vi "Drive for Time.vi"(8 "error in":errorcluster, 9 "Cluster":T6, 10 "Drivetrain":T1={"DevStatus"={"status"=FALSE, "code"=0, "source"=""}, "Motors[]"=[], "Square Inputs"=FALSE, "Max Output"=1.0}, 11 "Queue in":refnum<queue>) -> (0 "error out":errorcluster)   [LabVIEW 2016, in "Drive System.lvlib"]
uses:
  Drive System.lvlib
  DriveCmd.ctl
  DriveCmdList.ctl
  Varient Cmd Types/Drive Time.ctl
  <vilib>/Rock Robotics/WPI/RobotDrive/WPI_RobotDriveDevRef.ctl
  <vilib>/Rock Robotics/WPI/MotorControl/WPI_MotorControlDeviceRef.ctl
  <vilib>/Rock Robotics/WPI/MotorControl/WPI_MotorControlType.ctl
  <vilib>/Rock Robotics/SystemInterfaces/DIO/FPGA_DIOPWMChannel.ctl
  <vilib>/Rock Robotics/WPI/PWM/WPI_PWMDeadband.ctl
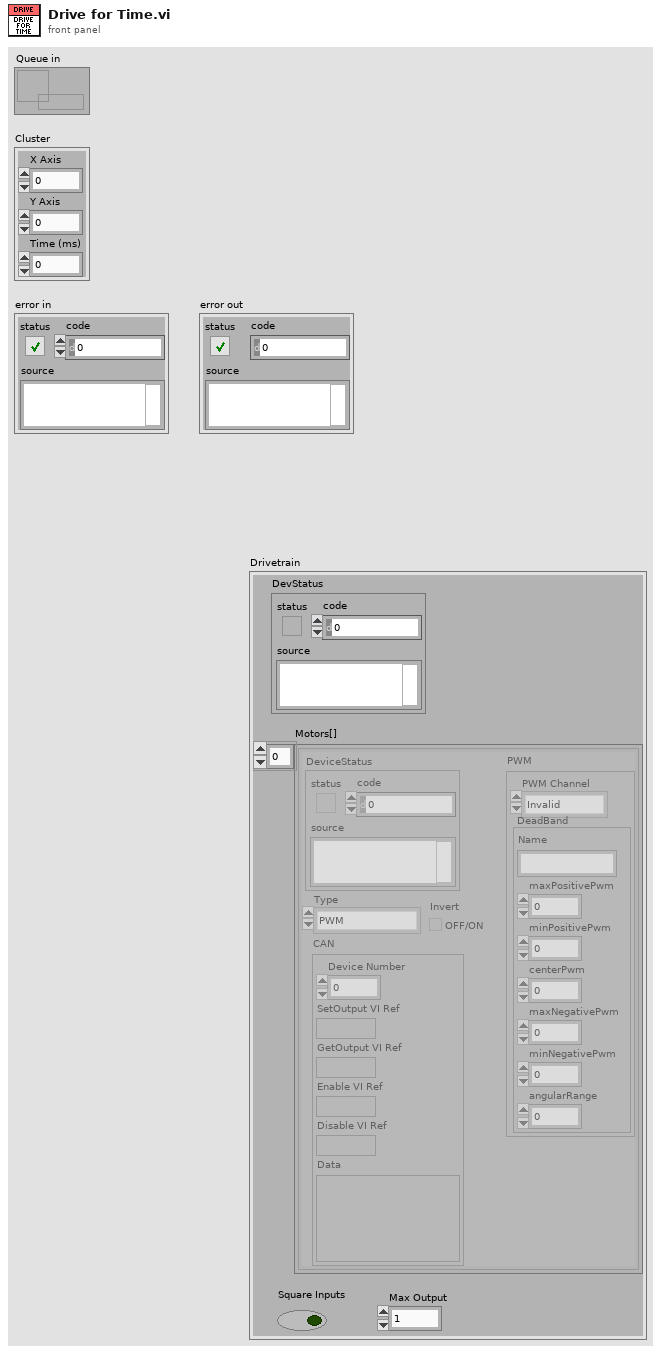
[diagram p1: front panel]
types:
  T1 = typedef "WPI_RobotDriveDevRef.ctl" = cluster{"DevStatus":errorcluster, "Motors[]":T2[], "Square Inputs":bool, "Max Output":dbl}
  T2 = typedef "WPI_MotorControlDeviceRef.ctl" = cluster{"DeviceStatus":errorcluster, "Type":T3, "PWM":cluster{"PWM Channel":T4, "DeadBand":T5}, "CAN":cluster{"Device Number":u8, "SetOutput VI Ref":variant, "GetOutput VI Ref":variant, "Enable VI Ref":variant, "Disable VI Ref":variant, "Data":variant}, "Invert":bool}
  T3 = typedef "WPI_MotorControlType.ctl" = enum16{"PWM", "CAN"}
  T4 = typedef "FPGA_DIOPWMChannel.ctl" = enum8{"PWM 0", "PWM 1", "PWM 2", "PWM 3", "PWM 4", "PWM 5", "PWM 6", "PWM 7", "PWM 8", "PWM 9", "PWM MXP 0", "PWM MXP 1", "PWM MXP 2", "PWM MXP 3", "PWM MXP 4", "PWM MXP 5", "PWM MXP 6", "PWM MXP 7", "PWM MXP 8", "PWM MXP 9", "Invalid"}
  T5 = typedef "WPI_PWMDeadband.ctl" = cluster{"Name":string, "maxPositivePwm":i32, "minPositivePwm":i32, "centerPwm":i32, "maxNegativePwm":i32, "minNegativePwm":i32, "angularRange":u16}
  T6 = typedef "Drive System.lvlib/Drive Time.ctl" = cluster{"X Axis":dbl, "Y Axis":dbl, "Time (ms)":u32}
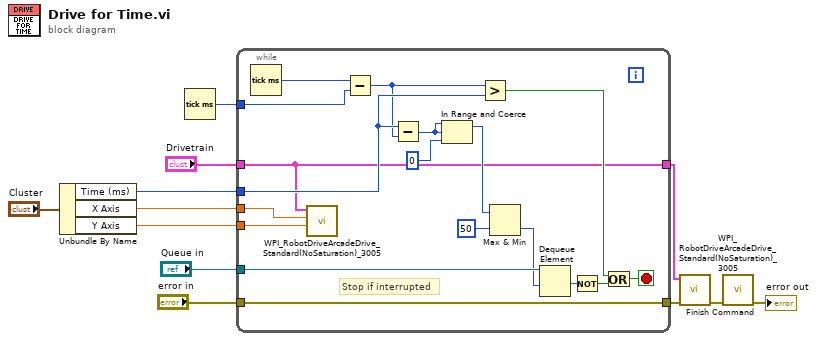
[diagram p0: block diagram]
diagram:
  n1 = Unbundle By Name("Cluster") -> ("Time (ms)"=w9:u32, "X Axis"=w8:dbl, "Y Axis"=w7:dbl)
  n2 = Tick Count (ms)() -> (millisecond timer value=w10:u32)
  n3 = while {
    tunnel: "Queue in" -> [w28]
    tunnel: w10 -> [w25]
    tunnel: w9 -> [w18]
    tunnel: w8 -> [w20]
    tunnel: w7 -> [w19]
    tunnel: "error in" -> [w21]
    tunnel: [w21] -> w3
    tunnel: "Drivetrain" -> [w13]
    tunnel: [w13] -> w1
    stop <- w27 stop-if-true
    # "Stop if interrupted"
    n4 = Tick Count (ms)() -> (millisecond timer value=w26:u32)
    n5 = call "WPI_RobotDriveArcadeDrive_Standard(NoSaturation)_3005.vi"("Y axis value"=w19, "X axis value"=w20, "RobotDriveDevRef"=w13) -> ()  [unwired: 7 in, 2 out]
    n6 = Subtract(x=w26, y=w25) -> (x-y=w16:u32)
    n7 = Subtract(x=w18, y=w16) -> (x-y=w14:u32)
    n8 = In Range and Coerce(upper limit=w14, x=w14, lower limit=u32 0) -> (coerced(x)=w15:u32)  [unwired: 1 out]
    n9 = Greater?(x=w16, y=w18) -> (0:w23:bool)
    n10 = Max & Min(x=w15, y=u32 50) -> (min(x,y)=w22:u32)  [unwired: 1 out]
    n11 = Dequeue Element(queue=w28, timeout in ms (-1)=w22) -> (timed out?=w30:bool)  [unwired: 1 in, 3 out]
    n12 = Not(x=w30) -> (.not. x?=w29:bool)
    n13 = Or(x=w23, y=w29) -> (x .or. y?=w27:bool)
  }
  n14 = call "WPI_RobotDriveArcadeDrive_Standard(NoSaturation)_3005.vi"("error in (no error)"=w3, "RobotDriveDevRef"=w1) -> ("error out"=w2:errorcluster)  [unwired: 8 in, 1 out]
  n15 = call "Finish Command.vi"("error in"=w2) -> ("error out"=→"error out":errorcluster)  [unwired: 10 in]
